vi "Change to Background Color.vi"(7 "change type":T1, 11 "item names":string[](array[string])) -> (3 "background colors":u32[](array[colorbox]))   [LabVIEW 2020, in "Ballard MIL-STD-1553 System Explorer.lvlib" / "Implementation.lvlib" / "Refresh.lvlib"]
uses:
  Refresh.lvlib
  Change Type.ctl
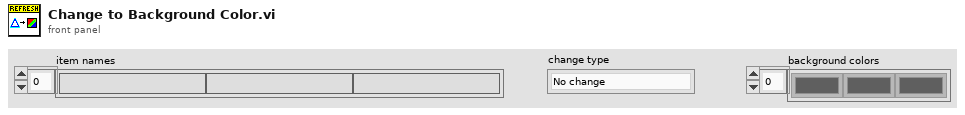
[diagram p1: front panel]
types:
  T1 = typedef "Ballard MIL-STD-1553 System Explorer.lvlib/Implementation.lvlib/Refresh.lvlib/Change Type.ctl" = enum16{"No change", "Modify", "Add", "Remove"}
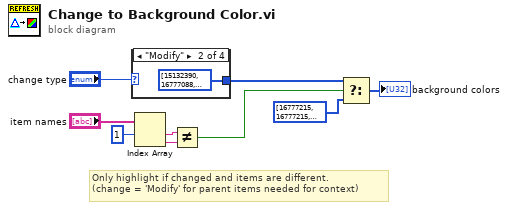
[diagram p0: block diagram]
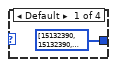
[diagram p2: hidden frame]
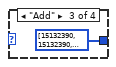
[diagram p3: hidden frame]
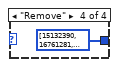
[diagram p4: hidden frame]
diagram:
  # "Only highlight if changed and items are different.\n(change = 'Modify' for parent items needed for context)"
  n1 = case shown="\"Modify\"" "change type" {
    tunnel: [u32[] [15132390, 15132390, 15132390] ("Bulk Cells:Background Colors") u32[] [15132390, 16777088, 16777088] ("Bulk Cells:Background Colors") u32[] [15132390, 15132390, 11468718] ("Bulk Cells:Background Colors") u32[] [15132390, 16761281, 15132390] ("Bulk Cells:Background Colors")] -> w3
    frame Default {
    }
    frame "Modify" {
    }
    frame "Add" {
    }
    frame "Remove" {
    }
  }
  n2 = Index Array(array="item names", index #1=1 ("index")) -> (element #1=w6:string, element #2=w7:string)  [unwired: 1 in]
  n3 = Not Equal?(x=w6, y=w7) -> (x != y?=w4:bool)
  n4 = Select(t=w3, s=w4, f=u32[] [16777215, 16777215, 16777215] ("Bulk Cells:Background Colors")) -> (s? t:f=→"background colors":u32[])
